vi "TDS DCPS Readback.vi"(8 "error in (no error)":errorcluster, 10 "Signal InstConfig":string, 11 "Address":string) -> (0 "error out":errorcluster, 3 "Readback Values":T1)   [LabVIEW 2025, in "Interface Functions.lvlib"]
uses:
  Interface Functions.lvlib
panel:
  # "DCPS Readback"
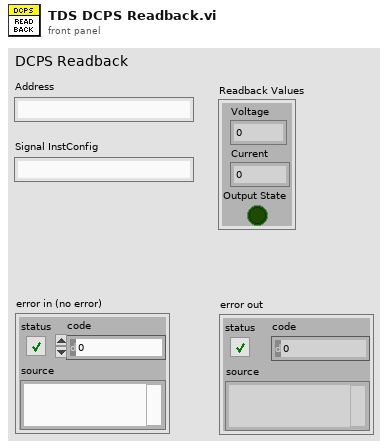
[diagram p1: front panel]
types:
  T1 = cluster{"Voltage":dbl, "Current":dbl, "Output State":bool}
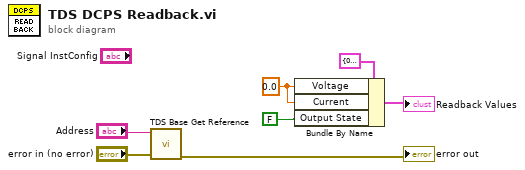
[diagram p0: block diagram]
diagram:
  w1 = 0.0 ("Voltage")
  n1 = call "TDS Base Get Reference.vi"("error in (no error)"="error in (no error)", "Address"="Address") -> ("error out"=→"error out":errorcluster)  [unwired: 8 in, 1 out]
  n2 = Bundle By Name(cluster=T1 {"Voltage"=0.0, "Current"=0.0, "Output State"=FALSE} ("Readback Values"), "Voltage"=w1, "Current"=w1, "Output State"=FALSE) -> (→"Readback Values":T1)
